vi "acquisition.vi"() -> ()   [LabVIEW 2025]
uses:
  <vilib>/measure/NI_MABase.lvlib
panel:
  in  "stop":bool
  in  "rapport cyclique (%)":dbl
  out "Waveform Graph":waveform(dbl)(graph)
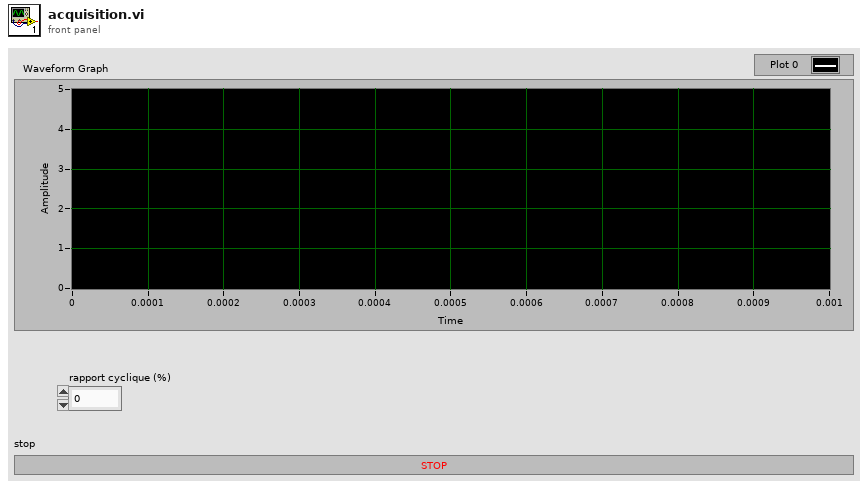
[diagram p1: front panel]
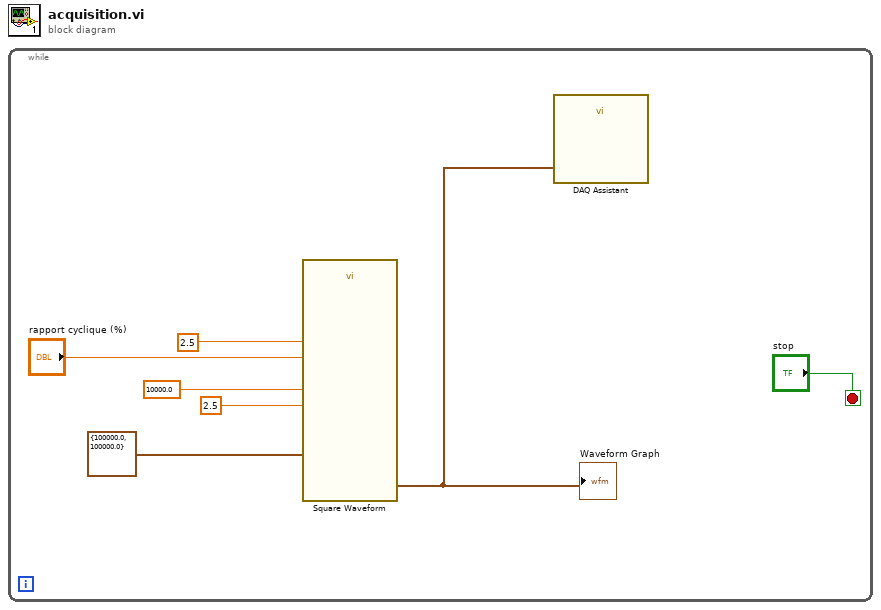
[diagram p0: block diagram]
diagram:
  n1 = while {
    stop <- "stop" stop-if-true
    n2 = call <vilib>:"Square Waveform.vi"("duty cycle (%)"="rapport cyclique (%)", "offset"=2.5, "sampling info"=cluster{"Fs":dbl, "#s":dbl} {"Fs"=100000.0, "#s"=100000.0}, "amplitude"=2.5, "frequency"=10000.0) -> ("signal out"=w1:waveform(dbl))  [unwired: 5 in, 1 out]
    "Waveform Graph" <- w1
    n3 = call "DAQ Assistant"("data"=w1) -> ()  [unwired: 16 in, 3 out]
  }
